vi "irsensorexample.vi"() -> ()   [LabVIEW 2022 SP3]
uses:
  <vilib>/Analysis/baseanly.llb/Mean (DBL).vi
  <vilib>/Analysis/NI_AALPro.lvlib
  <vilib>/Analysis/NI_AALBase.lvlib
panel:
  out "Voltage Samples Over Time":dbl(graph)
  in  "Sample Rate":dbl=1000.0
  in  "Number of Samples to Read":i32=100
  out "Filtered Signal from myDAQ":dynamicdata(graph) caption="Filtered Signal"
  in  "Cutoff Frequency":dbl=10.0 format="%0.4f"
  out "Average of Voltage Samples":dbl format="%0.2f"
  out "Raw Data from myDAQ":dynamicdata(graph)
  in  "stop (F)":bool
  out "Distance in centimeters":dbl(slide) scale=15.0..150.0
  # "cm"
  # "Setup: The top recessed frame has 3 fields, for the purpose of this example the Cutoff Frequency is set to 10 Hz, this frequency is used by the low pass filter to remove any stray spike that might occur.\nThe Sample Rate is the rate at which the each of the Number of Samples to Read are being read in at. The Number of Samples is the number of samples the myDAQ is told to acquire before returning data.\n\nAverage of Voltage Samples: This indicator shows the average of the samples being read in.\n\nVoltage Samples Over Time: Displays each set of sample's average value over time.\n\nRaw Data from myDAQ: Displays the sample set that is being retrieved.\n\nFiltered Signal from myDAQ: Displays the sample set after having the low pass filter applied\n\nDistance in centimeters: Displays the distance obtained after sending the average voltage into spline interpolation. The limits are set to 15cm to 150cm which are accurate limits of the infrared sensor."
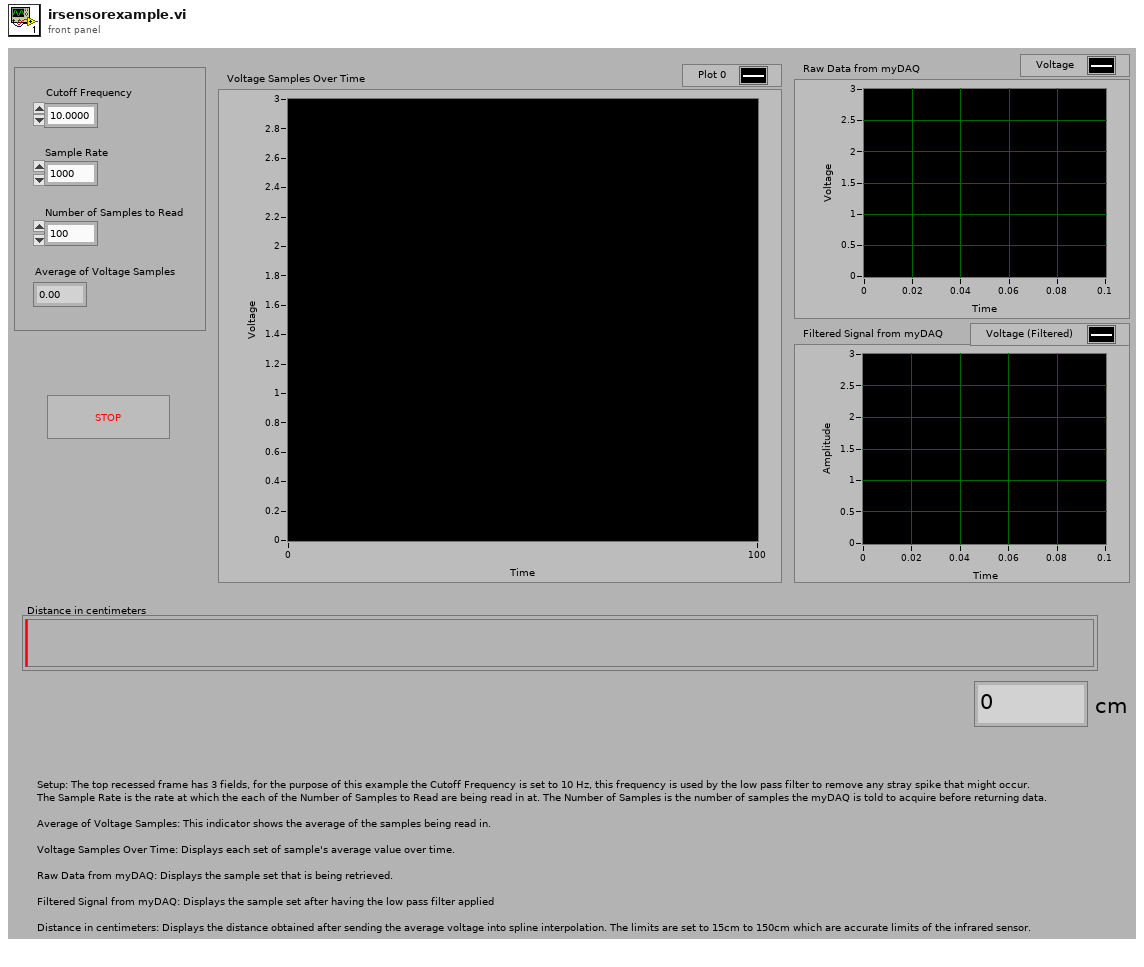
[diagram p1: front panel]
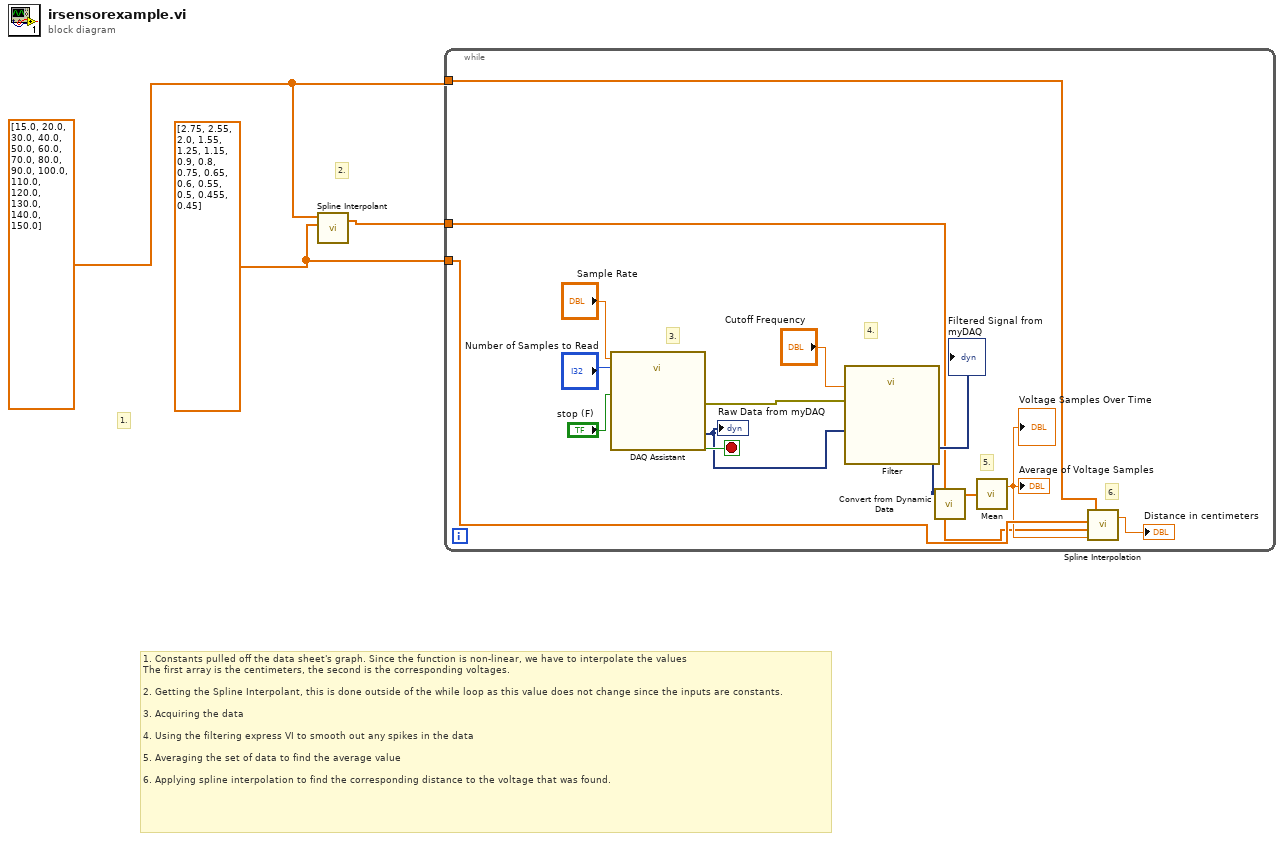
[diagram p0: block diagram]
diagram:
  w3 = dbl[] [15.0, 20.0, 30.0, 40.0, 50.0, 60.0, 70.0, 80.0, 90.0, 100.0, 110.0, 120.0, 130.0, 140.0, 150.0] ("Y")
  w2 = dbl[] [2.75, 2.55, 2.0, 1.55, 1.25, 1.15, 0.9, 0.8, 0.75, 0.65, 0.6, 0.55, 0.5, 0.455, 0.45] ("Y")
  # "2."
  # "1."
  # "1. Constants pulled off the data sheet's graph. Since the function is non-linear, we have to interpolate the values\nThe first array is the centimeters, the second is the corresponding voltages.\n\n2. Getting the Spline Interpolant, this is done outside of the while loop as this value does not change since the inputs are constants.\n\n3. Acquiring the data\n\n4. Using the filtering express VI to smooth out any spikes in the data\n\n5. Averaging the set of data to find the average value\n\n6. Applying spline interpolation to find the corresponding distance to the voltage that was found."
  n1 = call <vilib>:"Spline Interpolant.vi"("X"=w2, "Y"=w3) -> ("Interpolant"=w1:dbl[])  [unwired: 2 in, 1 out]
  n2 = while {
    tunnel: w3 -> [w14]
    tunnel: w2 -> [w13]
    tunnel: w1 -> [w4]
    stop <- w16 stop-if-true
    # "6."
    # "5."
    # "4."
    # "3."
    n3 = call "DAQ Assistant"("rate"="Sample Rate", "number of samples"="Number of Samples to Read", "stop (F)"="stop (F)") -> ("data"=w6:dynamicdata, "stopped"=w16:bool, "error out"=w10:errorcluster)  [unwired: 13 in, 1 out]
    "Raw Data from myDAQ" <- w6
    n4 = call "Filter"("error in (no error)"=w10, "Lower Cut-Off"="Cutoff Frequency", "Signal"=w6) -> ("Filtered Signal"=w7:dynamicdata)  [unwired: 7 in, 1 out]
    "Filtered Signal from myDAQ" <- w7
    n5 = call "Convert from Dynamic Data"("Dynamic Data Type"=w7) -> ("Array"=w8:dbl[])  [unwired: 3 in]
    n6 = call-poly <vilib>:"Mean.vi"("X"=w8) -> ("mean"=w5:dbl)  [unwired: 1 out]
    "Average of Voltage Samples" <- w5
    "Voltage Samples Over Time" <- w5
    n7 = call <vilib>:"Spline Interpolation.vi"("x value"=w5, "Interpolant"=w4, "X"=w13, "Y"=w14) -> ("interpolation value"=→"Distance in centimeters":dbl)  [unwired: 1 out]
  }
